vi "Actor Core.vi"(8 "error in":errorcluster, 11 "SCADA in":refnum<class "EMS.lvclass">) -> (0 "error out":errorcluster, 3 "Actor out":refnum<class "Actor.lvclass">)   [LabVIEW 2018, in "EMS Core.lvlib" / "EMS.lvclass"]
doc: "(<B>Filename</B>: Actor Framework.lvlib:Actor.lvclass:Actor Core.vi)\n\nReceives messages to the actor, reacts to them, and initiates any error handling that may shut the actor down.\n\nDescendant classes may override this VI to append parallel tasks for the actor to complete while it handles messages. Overrides use the Call Parent Method node."
uses:
  EMS.lvclass
  C:/Program Files (x86)/National Instruments/LabVIEW 2018/vi.lib/ActorFramework/Actor/Actor.lvclass
  C:/Users/Administrator/Desktop/LabVIEW EMS/EMS Generic Actor/EMS Generic/EMS Generic.lvclass
  <vilib>/ActorFramework/Actor/Actor.lvclass
  IED Actors/IED Actor/IED Messages/Watchdog Reset Msg/Watchdog Reset Msg.lvclass
  C:/Program Files (x86)/National Instruments/LabVIEW 2018/vi.lib/ActorFramework/Message/Message.lvclass
  <vilib>/ActorFramework/Message Enqueuer/Message Priority.ctl
  Device Specific Actors/AE75TX Actor/AE75TX/AE75TX.lvclass
  EMS.lvclass/EMS.ctl
  <vilib>/ActorFramework/Actor/Actor.lvclass/Actor.ctl
  EMS Generic Actor/EMS Generic/EMS Generic.lvclass/EMS Generic.ctl
  <vilib>/ActorFramework/Message Enqueuer/Message Enqueuer.lvclass/Message Enqueuer.ctl
  EMS Messages/Return DeviceID Array Msg/Return DeviceID Array Msg.lvclass/Return DeviceID Array Msg.ctl
  <vilib>/ActorFramework/Message Enqueuer/Init from Existing Queue.vi
  <vilib>/ActorFramework/Message Enqueuer/Enqueue.vi
  EMS Messages/Device Discovery Init Msg/Device Discovery Init Msg.lvclass
  EMS Messages/Return DeviceID Array Msg/Return DeviceID Array Msg.lvclass
  <vilib>/ActorFramework/Message Priority Queue/Priority Enqueue.vi
  <vilib>/ActorFramework/Message Enqueuer/Message Enqueuer.lvclass
  EMS Generic Actor/EMS Generic/EMS Generic.lvclass
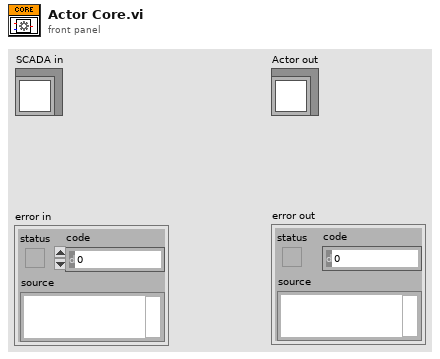
[diagram p1: front panel]
types:
  T1 = typedef "Actor Framework.lvlib/Message Enqueuer.lvclass/Message Priority.ctl" = enum16{"Low", "Normal", "High"}
  T2 = typedef "EMS Generic Actor.lvlib/EMS Generic.lvclass/EMS Generic User Events.ctl" = cluster{"stop":refnum<user-event>}
  T3 = typedef "EMS Generic Actor.lvlib/EMS Generic.lvclass/Data Type DVRs.ctl" = cluster{"IED_Status":refnum<data-value>, "IED_Status_0":refnum<data-value>, "DER_Measurement":refnum<data-value>, "DER_Info":refnum<data-value>, "DER_Status":refnum<data-value>, "ES_Measurement":refnum<data-value>, "ES_Info":refnum<data-value>, "PV_Info":refnum<data-value>, "SmartRelay_Info":refnum<data-value>, "SmartRelay_Measurement":refnum<data-value>, "Meter_Info":refnum<data-value>, "Meter_Measurement":refnum<data-value>, "HVAC_Status":refnum<data-value>, "HVAC_Measurement":refnum<data-value>, "PriceData_RealTime":refnum<data-value>, "PriceData_Demand":refnum<data-value>, "PriceData_Energy":refnum<data-value>, "ForecastData_Long":refnum<data-value>, "ForecastData_Short":refnum<data-value>, "DER_Control":refnum<data-value>, "DER_SetPointF":refnum<data-value>, "DER_SetPointP":refnum<data-value>, "DER_SetPointQ":refnum<data-value>, "DER_SetPointPF":refnum<data-value>, "DER_SetPointV":refnum<data-value>, "PV_setCurtailment":refnum<data-value>, "PV_setRampRate":refnum<data-value>, "Relay_Control":refnum<data-value>, "Load_Control":refnum<data-value>, "HVAC_Control":refnum<data-value>, "Generator_Info":refnum<data-value>, "ForecastData_Long_Backup":refnum<data-value>, "PriceData_RealTime_Backup":refnum<data-value>}
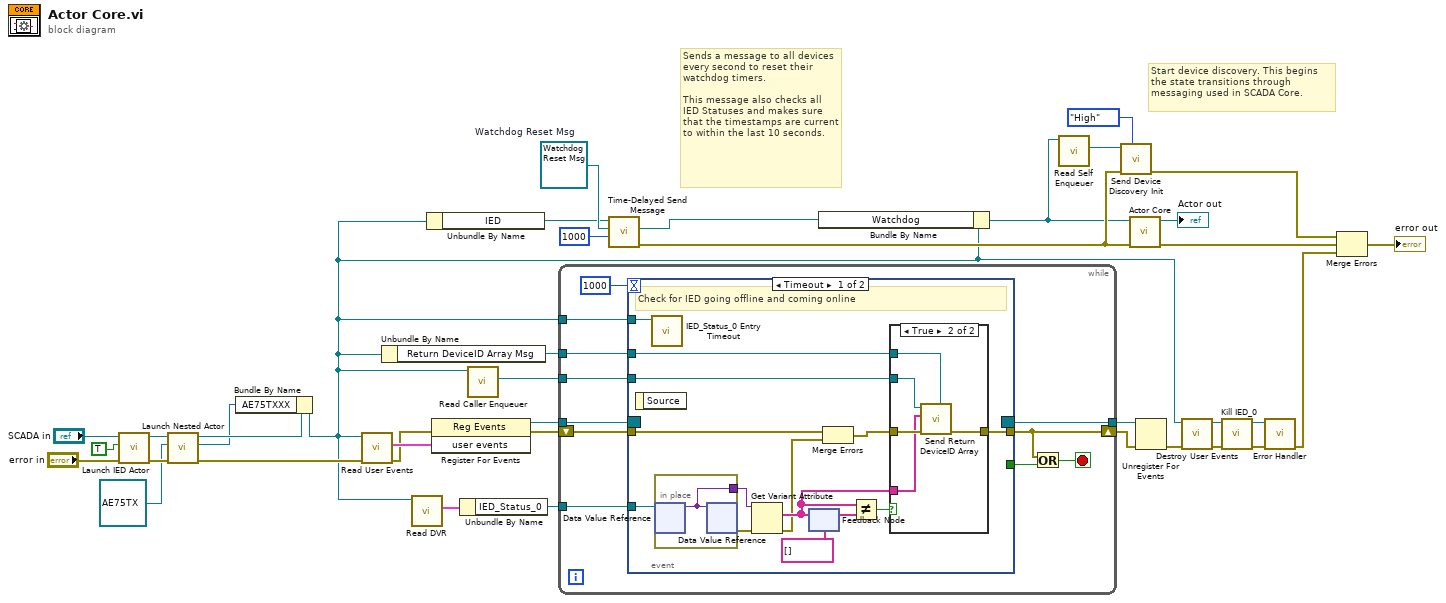
[diagram p0: block diagram]
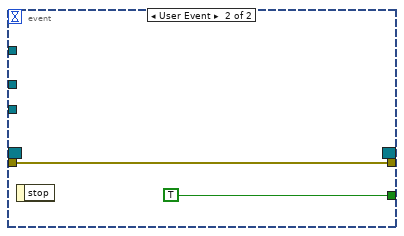
[diagram p3: hidden frame]
diagram:
  w32 = refnum<class "Watchdog Reset Msg.lvclass"> refnum  # Watchdog Reset Msg
  # "Start device discovery. This begins the state transitions through messaging used in SCADA Core."
  # "Sends a message to all devices every second to reset their watchdog timers.\n\nThis message also checks all IED Statuses and makes sure that the timestamps are current to within the last 10 seconds."
  n1 = call "Launch IED Actor.vi"("error in"="error in", "Discovery Mode? (F)"=TRUE, "SCADA in"="SCADA in") -> ("error out"=w5:errorcluster, "SCADA out"=w7:refnum<class "EMS.lvclass">)  [unwired: 7 in]
  n2 = call <vilib>:"Launch Nested Actor.vi"("error in (no error)"=w5, "Nested Actor"=refnum<class "AE75TX.lvclass"> refnum ("AE75TX Actor.lvlib:AE75TX"), "Caller Actor in"=w7) -> ("error out"=w4:errorcluster, "Nested Actor's Enqueuer"=w2:refnum<class "Message Enqueuer.lvclass">, "Caller Actor out"=w6:refnum<class "EMS.lvclass">)  [unwired: 6 in]
  n3 = Bundle By Name(cluster=w6, "AE75TXXX"=w2) -> (w3:refnum<class "EMS.lvclass">)
  n4 = call "Read User Events.vi"("error in (no error)"=w4, "EMS Generic in"=w3) -> ("error out"=w19:errorcluster, "user events"=w27:T2)  [unwired: 7 in, 1 out]
  n5 = Unbundle By Name(w3) -> ("Return DeviceID Array Msg"=w15:refnum<class "Return DeviceID Array Msg.lvclass">)
  n6 = call "Read DVR.vi"("EMS Generic in"=w3) -> ("DVR"=w24:T3)  [unwired: 9 in, 1 out]
  n7 = Unbundle By Name(w3) -> ("IED"=w28:refnum<class "Message Enqueuer.lvclass">)
  n8 = register-events(error in=w19, w27) -> (reference out=w26:refnum<event-registration>, error out=w18:errorcluster)  [unwired: 1 in]
  n9 = Unbundle By Name(w24) -> ("IED_Status_0"=w23:refnum<data-value>)
  n10 = call <vilib>:"Read Caller Enqueuer.vi"("Actor"=w3) -> ("Caller Enqueuer"=w14:refnum<class "Message Enqueuer.lvclass">)  [unwired: 10 in]
  n11 = while {
    tunnel: w26 -> [w49]
    tunnel: w23 -> [w47]
    tunnel: [w46] -> w22
    shift-right: [w42] -> w17
    shift-left: w18 -> [w43]
    tunnel: w15 -> [w45]
    tunnel: w14 -> [w44]
    tunnel: w3 -> [w39]
    stop <- w40 stop-if-true
    n12 = event shown="[0] Timeout" {
      selector: w49 -> [_ _]
      dyn-events: [_ _] -> w46
      timeout: 1000 -> [_ _]
      tunnel: [_ TRUE] -> w41
      tunnel: w47 -> [w63 _]
      tunnel: w45 -> [w62 _]
      tunnel: w44 -> [w61 _]
      tunnel: w43 -> [w60 w71]
      tunnel: [w59 w71] -> w42
      tunnel: w39 -> [w51 _]
      event Timeout {
        # "Check for IED going offline and coming online"
        n13 = event-data() -> ()  [unwired: 1 in, 1 out]
        n14 = call "IED_Status_0 Entry Timeout.vi"("SCADA in"=w51) -> ()  [unwired: 11 in]
        n15 = in-place {
          in-place-border: [w70] -> w55
          n16 = in-place-dvr #1(w63) -> (w70:variant)  [unwired: 1 out]
          n17 = in-place-dvr #1(w70) -> (w53:errorcluster)  [unwired: 1 out]
        }
        n18 = Get Variant Attribute(Variant=w55, error in=w53) -> (names=w54:string[], error out=w52:errorcluster)  [unwired: 2 in, 2 out]
        n19 = feedback-in #2(w54) -> ()
        n20 = feedback #2(string[] []) -> (w57:string[])
        n21 = Merge Errors(w60, w52) -> (w58:errorcluster)
        n22 = Not Equal?(x=w54, y=w57) -> (x != y?=w56:bool)
        n23 = case shown="True" w56 {
          tunnel: w62 -> [_ w69]
          tunnel: w61 -> [_ w68]
          tunnel: [w64 w67] -> w59
          tunnel: w58 -> [w64 w66]
          tunnel: w54 -> [_ w65]
          frame False {
          }
          frame True {
            n24 = call "Send Return DeviceID Array.vi"("Message Type"=w69, "error in (no error)"=w66, "DeviceID Array"=w65, "Message Enqueuer"=w68) -> ("error out"=w67:errorcluster)  [unwired: 6 in, 1 out]
          }
        }
      }
      event User Event {
        n25 = event-data() -> ()  [unwired: 1 in, 1 out]
      }
    }
    n26 = Or(x=w42, y=w41) -> (x .or. y?=w40:bool)
  }
  n27 = call <vilib>:"Time-Delayed Send Message.vi"("Milliseconds To Wait"=1000, "Message"=w32, "Message Enqueuer"=w28) -> ("error out"=w33:errorcluster, "Delivery Notifier"=w31:refnum<notifier>)  [unwired: 7 in]
  n28 = Bundle By Name(cluster=w3, "Watchdog"=w31) -> (w29:refnum<class "EMS.lvclass">)
  n29 = call <vilib>:"Read Self Enqueuer.vi"("Actor"=w29) -> ("Self Enqueuer"=w36:refnum<class "Message Enqueuer.lvclass">)  [unwired: 10 in]
  n30 = call "Send Device Discovery Init.vi"("Message Priority (Normal)"=Message_Priority."High", "error in (no error)"=w33, "Message Enqueuer"=w36) -> ("error out"=w35:errorcluster)  [unwired: 7 in, 1 out]
  n31 = call-parent "Actor Core.vi"("error in"=w33, "Actor in"=w29) -> ("error out"=w38:errorcluster, "Actor out"=→"Actor out":refnum<class "Actor.lvclass">)  [unwired: 8 in]
  n32 = Unregister For Events(event registration refnum=w22, error in=w17) -> (error out=w16:errorcluster)
  n33 = call-dynamic "Destroy User Events.vi"("error in"=w16, "EMS Generic in"=w3) -> ("error out"=w12:errorcluster, "EMS Generic out"=w13:refnum<class "EMS.lvclass">)  [unwired: 8 in]
  n34 = call "Kill IED_0.vi"("error in"=w12, "SCADA in"=w13) -> ("error out"=w10:errorcluster, "SCADA out"=w11:refnum<class "EMS.lvclass">)  [unwired: 8 in]
  n35 = call-dynamic "Error Handler.vi"("error in"=w10, "EMS Generic in"=w11) -> ("error out"=w9:errorcluster)  [unwired: 8 in, 1 out]
  n36 = Merge Errors(w35, w38, w9) -> (→"error out":errorcluster)
